vi "Read History.vi"(8 "error in (no error)":errorcluster, 11 "Optimiser Cell in":refnum<class "Optimiser Cell.lvclass">) -> (0 "error out":errorcluster, 2 "History":T1[](array[typedef]), 3 "Optimiser Cell out":refnum<class "Optimiser Cell.lvclass">)   [LabVIEW 2020, in "CIRCUS_uServices.lvlib" / "Run Utilities.lvlib" / "Optimiser Cell.lvclass"]
uses:
  Optimiser Cell.lvclass
  Name with value pair.ctl
  Analysis Framework/Analysis Framework.lvclass
  Optimiser Results.ctl
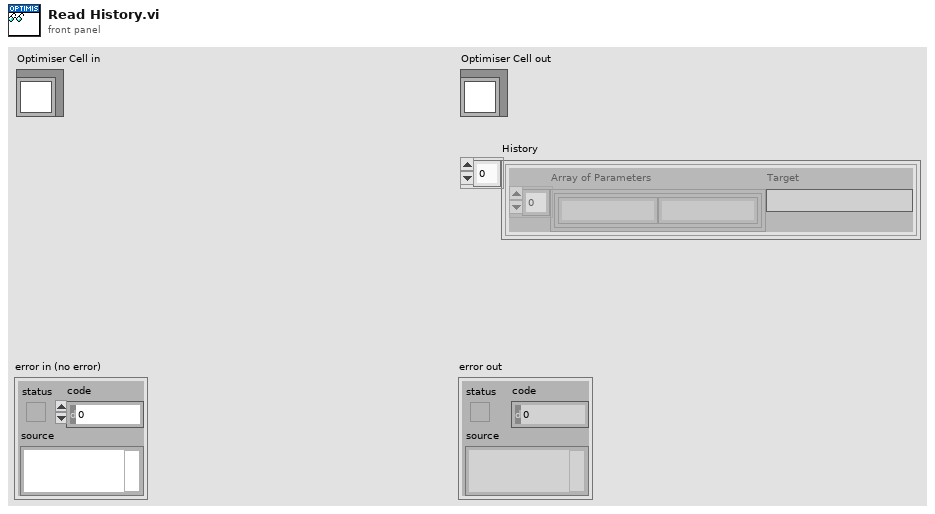
[diagram p1: front panel]
types:
  T1 = typedef "CIRCUS_uServices.lvlib/Run Utilities.lvlib/Optimiser Cell.lvclass/Optimiser Results.ctl" = cluster{"Array of Parameters":T2[], "Target":string}
  T2 = typedef "CIRCUS_uServices.lvlib/Analysis Framework.lvclass/Name with value pair.ctl" = cluster{"Name":string, "Value":string}
  T3 = typedef "Run Utilities.lvlib/Optimiser Cell.lvclass/Optimiser Results.ctl" = cluster{"Array of Parameters":T4[], "Target":string}
  T4 = typedef "Analysis Framework.lvclass/Name with value pair.ctl" = cluster{"Name":string, "Value":string}
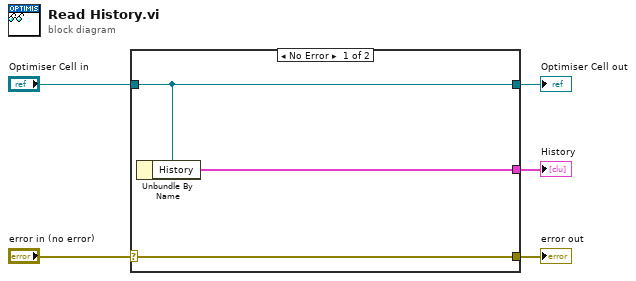
[diagram p0: block diagram]
diagram:
  n1 = case shown="No Error" "error in (no error)" {
    selector: "error in (no error)" -> [w8 w9]
    tunnel: [w8 w9] -> w4
    tunnel: [w7 w10] -> w2
    tunnel: "Optimiser Cell in" -> [w7 w10]
    tunnel: [w6 _] -> w1
    frame No Error {
      n2 = Unbundle By Name(w7) -> ("History"=w6:T3[])
    }
    frame Error {
    }
  }
  "error out" <- w4
  "Optimiser Cell out" <- w2
  "History" <- w1
